vi "CacheConfigFile-SMTPAuthentication.vi"() -> (2 "Authentication Credentials":T1)   [LabVIEW 2016]
uses:
  SMTPCredentials.ctl
  Anemometry Sub Vis/Globals/Constants_global.vi
  <vilib>/Utility/config.llb/Read Key (String).vi
  <vilib>/Utility/config.llb/Write Key (String).vi
  <vilib>/Utility/config.llb/NI_LVConfig.lvlib
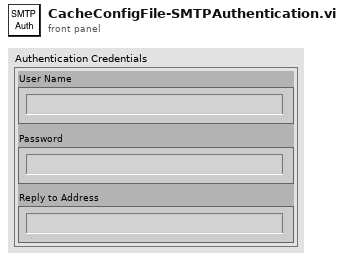
[diagram p1: front panel]
types:
  T1 = typedef "SMTPCredentials.ctl" = cluster{"User Name":string, "Password":string, "Reply to Address":string}
  T2 = typedef "NI_LVConfig.lvlib/Config Data RefNum.ctl" = refnum<k1>
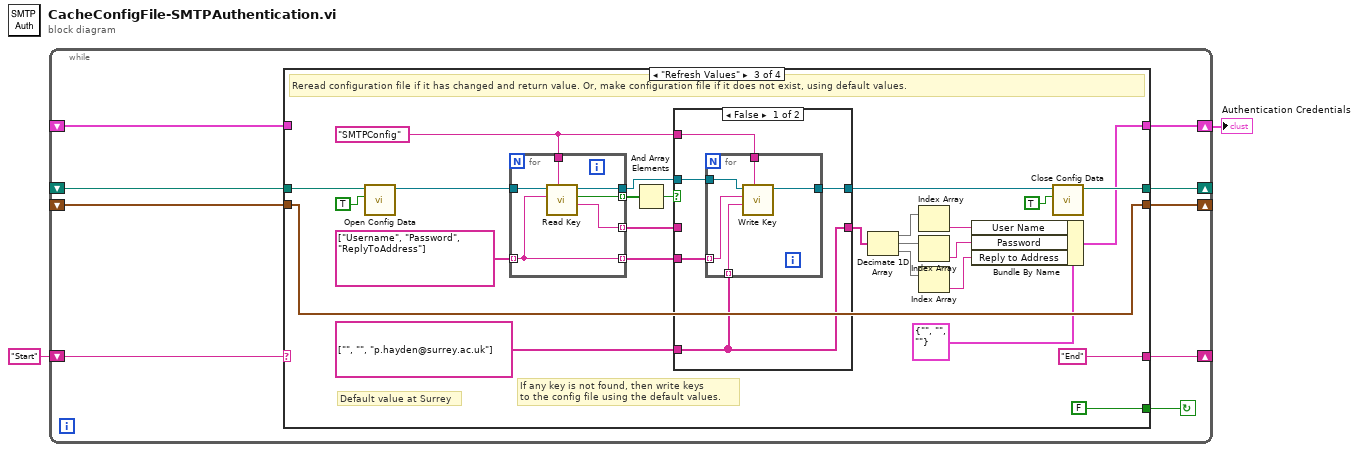
[diagram p0: block diagram]
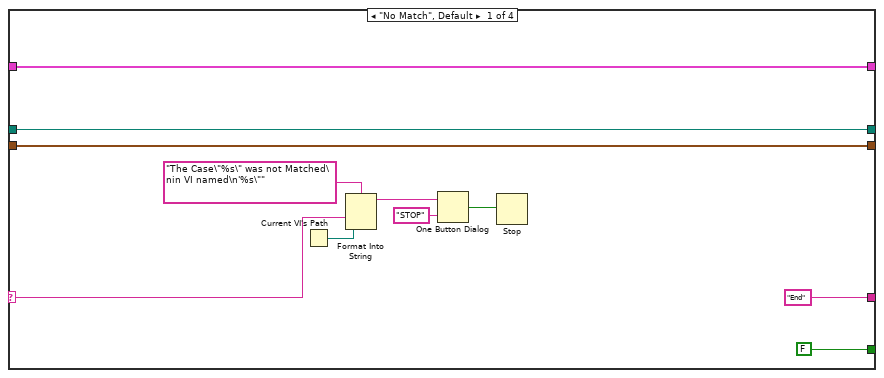
[diagram p2: hidden frame]
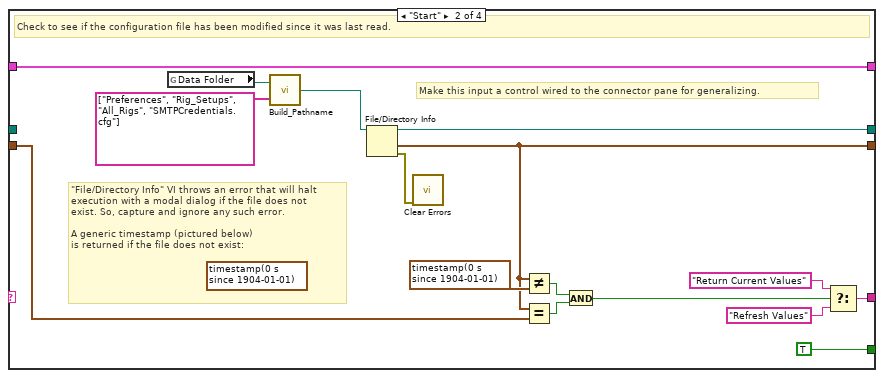
[diagram p3: hidden frame]
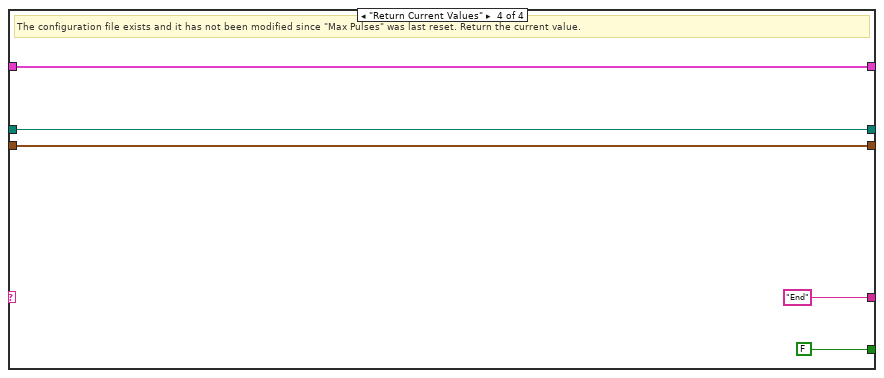
[diagram p5: hidden frame]
diagram:
  n1 = while {
    shift-left: _ -> [w5]
    shift-right: [w7] -> _
    shift-left: _ -> [w6]
    shift-right: [w8] -> w1
    shift-left: "Start" -> [w9]
    shift-right: [w10] -> _
    shift-right: [w4] -> _
    shift-left: _ -> [w3]
    stop <- w11 continue-if-true
    n2 = case shown="\"Refresh Values\"" w9 {
      selector: w9 -> [w13 _ _ _]
      tunnel: [FALSE TRUE FALSE FALSE] -> w11
      tunnel: ["End" w34 "End" "End"] -> w10
      tunnel: [w15 w37 w41 w87] -> w8
      tunnel: [w14 w31 w57 w86] -> w7
      tunnel: w6 -> [w15 w37 _ w87]
      tunnel: w5 -> [w14 w33 w57 w86]
      tunnel: [w12 w27 w58 w83] -> w4
      tunnel: w3 -> [w12 _ w59 w83]
      frame "No Match", Default {
        n3 = Current VI's Path() -> (path=w17:path)
        n4 = Format Into String(format string="The Case\"%s\" was not Matched\nin VI named\n'%s\"" ("Format String"), w13, w17) -> (resulting string=w20:string)  [unwired: 2 in, 1 out]
        n5 = One Button Dialog(message=w20, button name ("OK")="STOP") -> (true=w18:bool)
        n6 = Stop(stop? (T)=w18) -> ()
      }
      frame "Start" {
        (unwired) "Return Current Values"
        (unwired) timestamp(0 s since 1904-01-01) ("last mod")
        # "Make this input a control wired to the connector pane for generalizing."
        # "Check to see if the configuration file has been modified since it was last read."
        # "\"File/Directory Info\" VI throws an error that will halt execution with a modal dialog if the file does not \nexist. So, capture and ignore any such error.\n\nA generic timestamp (pictured below) is returned if the file does not exist:"
        # "\"File/Directory Info\" VI throws an error that will halt execution with a modal dialog if the file does not \nexist. So, capture and ignore any such error.\n\nA generic timestamp (pictured below)\nis returned if the file does not exist:"
        # "\"File/Directory Info\" VI throws an error that will halt execution with a modal dialog if the file does not \nexist. So, capture and ignore any such error.\n\nA generic timestamp (pictured below)\nis returned if the file does not exist:"
        n7 = global read "Constants_global.vi" "Data Folder"() -> (w25:path)
        n8 = call "Build_Pathname.vi"("PathElements"=string[] ["Preferences", "Rig_Setups", "All_Rigs", "SMTPCredentials.cfg"], "PathnameIn"=w25) -> ("AppendedPath"=w24:path)
        n9 = File/Directory Info(path=w24) -> (path out=w27:path, last mod=w31:timestamp, error out=w38:errorcluster)  [unwired: 1 in, 4 out]
        n10 = call <vilib>:"Clear Errors.vi"("error in (no error)"=w38) -> ()  [unwired: 5 in, 2 out]
        n11 = Not Equal?(x=w31, y=timestamp(0 s since 1904-01-01) ("last mod")) -> (x != y?=w30:bool)
        n12 = Equal?(x=w31, y=w33) -> (x = y?=w29:bool)
        n13 = And(x=w30, y=w29) -> (x .and. y?=w35:bool)
        n14 = Select(t="Return Current Values", s=w35, f="Refresh Values") -> (s? t:f=w34:string)
      }
      frame "Refresh Values" {
        w55 = "SMTPConfig" ("section")
        # "If any key is not found, then write keys\nto the config file using the default values."
        # "Default value at Surrey"
        # "Reread configuration file if it has changed and return value. Or, make configuration file if it does not exist, using default values."
        n15 = call <vilib>:"Open Config Data.vi"("create file if necessary (T)"=TRUE, "configuration file path"=w59) -> ("refnum"=w62:T2)  [unwired: 7 in, 2 out]
        n16 = for {
          tunnel: w62 -> [w70]
          tunnel: w55 -> [w69]
          tunnel: string[] ["Username", "Password", "ReplyToAddress"] -> [w65] mode=indexing
          tunnel: [w68] -> w50
          tunnel: [w67] -> w53 mode=indexing
          tunnel: [w66] -> w51 mode=indexing
          tunnel: [w65] -> w39 mode=indexing
          n17 = call-poly <vilib>:"Read Key.vi"("section"=w69, "key"=w65, "refnum"=w70) -> ("value"=w66:string, "found?"=w67:bool, "refnum out"=w68:T2)  [unwired: 5 in, 1 out]
        }
        n18 = And Array Elements(Boolean array=w53) -> (logical AND=w52:bool)
        n19 = case shown="False" w52 {
          tunnel: w55 -> [w74 _]
          tunnel: [w71 w81] -> w60
          tunnel: w51 -> [_ w82]
          tunnel: [w72 w82] -> w49
          tunnel: w50 -> [w75 w81]
          tunnel: string[] ["", "", "p.hayden@surrey.ac.uk"] -> [w72 _]
          tunnel: w39 -> [w73 _]
          frame False {
            n20 = for {
              tunnel: [w80] -> w71
              tunnel: w75 -> [w79]
              tunnel: w74 -> [w78]
              tunnel: w73 -> [w77] mode=indexing
              tunnel: w72 -> [w76] mode=indexing
              n21 = call-poly <vilib>:"Write Key.vi"("section"=w78, "value"=w76, "key"=w77, "refnum"=w79) -> ("refnum out"=w80:T2)  [unwired: 5 in, 2 out]
            }
          }
          frame True {
          }
        }
        n22 = Decimate 1D Array(w49) -> (w46:string[], w47:string[], w45:string[])
        n23 = Index Array(array=w46) -> (element=w43:string)  [unwired: 1 in]
        n24 = Index Array(array=w47) -> (element=w44:string)  [unwired: 1 in]
        n25 = Index Array(array=w45) -> (element=w42:string)  [unwired: 1 in]
        n26 = Bundle By Name(cluster=T1 {"User Name"="", "Password"="", "Reply to Address"=""} ("Authentication Credentials"), "User Name"=w43, "Password"=w44, "Reply to Address"=w42) -> (w41:T1)
        n27 = call <vilib>:"Close Config Data.vi"("write file if changed (T)"=TRUE, "refnum"=w60) -> ("file path"=w58:path)  [unwired: 8 in, 1 out]
      }
      frame "Return Current Values" {
        # "The configuration file exists and it has not been modified since \"Max Pulses\" was last reset. Return the current value."
      }
    }
  }
  "Authentication Credentials" <- w1
